vi "三维图像.vi"() -> ()   [LabVIEW 2023]
panel:
  in  "Path":path
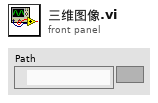
[diagram p1: front panel]
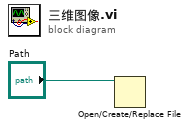
[diagram p0: block diagram]
diagram:
  n1 = Open/Create/Replace File(file path (use dialog)="Path") -> ()  [unwired: 5 in, 3 out]
